vi "_Read RT Table.vi"(4 "error in (no error)":errorcluster, 6 "key":string) -> (0 "error out":errorcluster, 1 "Table":dbl[][](array[numeric]))   [LabVIEW 2012]
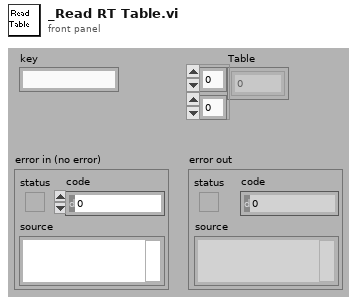
[diagram p1: front panel]
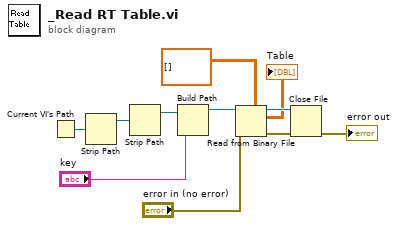
[diagram p0: block diagram]
diagram:
  n1 = Current VI's Path() -> (path=w9:path)
  n2 = Strip Path(path=w9) -> (stripped path=w10:path)  [unwired: 1 out]
  n3 = Strip Path(path=w10) -> (stripped path=w11:path)  [unwired: 1 out]
  n4 = Build Path(base path=w11, name or relative path="key") -> (appended path=w7:path)
  n5 = Read from Binary File(5:dbl[][] [], 8:"error in (no error)", 11:w7) -> (0:w5:errorcluster, 2:→"Table":dbl[][], 3:w4:refnum<file>)  [unwired: 4 out]
  n6 = Close File(refnum=w4, error in=w5) -> (error out=→"error out":errorcluster)  [unwired: 1 out]
